vi "SinglePreview.vi"(8 "error in (no error)":errorcluster, 11 "Avantes in":refnum<class "Avantes.lvclass">) -> (0 "error out":errorcluster, 1 "Data Raw":T1(array[cluster]), 2 "Data":T1(array[cluster]), 3 "Avantes out":refnum<class "Avantes.lvclass">, 4 "Darkspec":T1(array[cluster]))   [LabVIEW 2020, in "Avantes.lvclass"]
uses:
  <instrlib>/Classes/CCD/Avantes/Avantes.lvclass
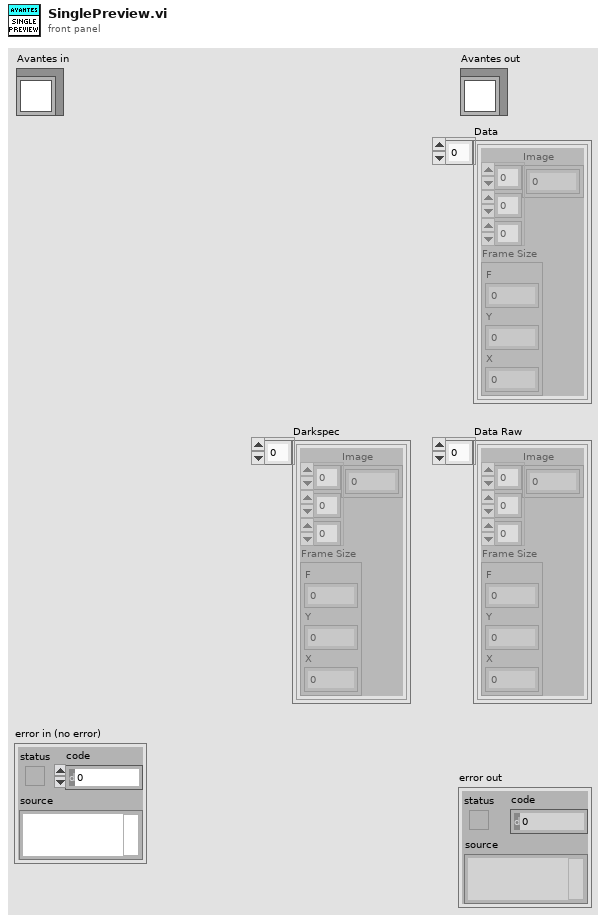
[diagram p1: front panel]
types:
  T1 = cluster{"Image":dbl[][][], "Frame Size":cluster{"F":i32, "Y":i32, "X":i32}}[]
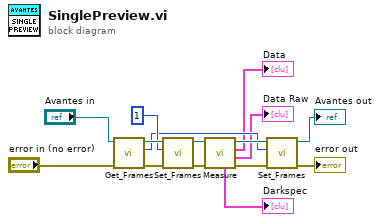
[diagram p0: block diagram]
diagram:
  n1 = call-dynamic "Get_Frames.vi"("error in (no error)"="error in (no error)", "Avantes in"="Avantes in") -> ("error out"=w12:errorcluster, "Frames"=w5:i32, "Avantes out"=w13:refnum<class "Avantes.lvclass">)  [unwired: 7 in]
  n2 = call-dynamic "Set_Frames.vi"("error in (no error)"=w12, "Frames"=1, "Avantes in"=w13) -> ("error out"=w9:errorcluster, "Avantes out"=w10:refnum<class "Avantes.lvclass">)  [unwired: 7 in]
  n3 = call-dynamic "Measure.vi"("error in (no error)"=w9, "Avantes in"=w10) -> ("error out"=w6:errorcluster, "Data Raw"=→"Data Raw":T1, "Data"=→"Data":T1, "Avantes out"=w7:refnum<class "Avantes.lvclass">, "Darkspec"=→"Darkspec":T1)  [unwired: 3 in, 2 out]
  n4 = call-dynamic "Set_Frames.vi"("error in (no error)"=w6, "Frames"=w5, "Avantes in"=w7) -> ("error out"=→"error out":errorcluster, "Avantes out"=→"Avantes out":refnum<class "Avantes.lvclass">)  [unwired: 7 in]
